vi "BuildArraySampleImages.vi"(11 "chaîne":string) -> (3 "3DArray":cluster{"Tableau":string[][]}[](array[cluster]))   [LabVIEW 2020]
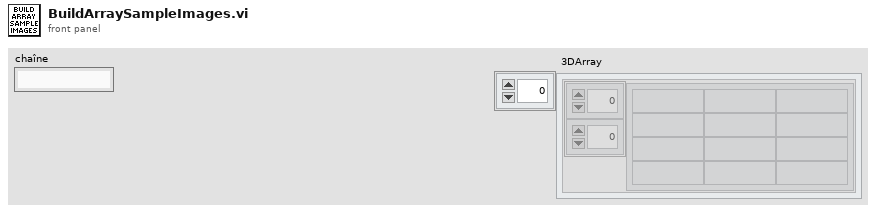
[diagram p1: front panel]
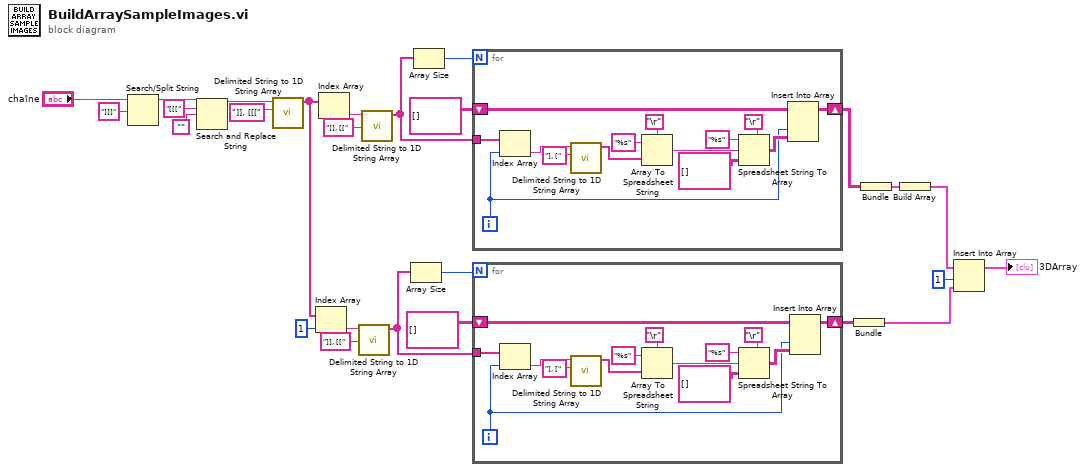
[diagram p0: block diagram]
diagram:
  n1 = Search/Split String(string="chaîne", search string/char (-)="]]]" ("chaîne/car. recherché (-)")) -> (substring before match=w25:string)  [unwired: 1 in, 2 out]
  n2 = Search and Replace String(input string=w25, search string="[[[" ("chaîne recherchée"), replace string="") -> (result string=w22:string)  [unwired: 5 in, 3 out]
  n3 = call <vilib>:"Delimited String to 1D String Array.vi"("delimiter"="]], [[[", "delimited string"=w22) -> ("string array"=w11:string[])  [unwired: 9 in]
  n4 = Index Array(array=w11, index=1 ("indice")) -> (element=w16:string)
  n5 = Index Array(array=w11) -> (element=w19:string)  [unwired: 1 in]
  n6 = call <vilib>:"Delimited String to 1D String Array.vi"("delimiter"="]], [[", "delimited string"=w16) -> ("string array"=w13:string[])  [unwired: 9 in]
  n7 = call <vilib>:"Delimited String to 1D String Array.vi"("delimiter"="]], [[", "delimited string"=w19) -> ("string array"=w18:string[])  [unwired: 9 in]
  n8 = Array Size(array=w13) -> (size(s)=w10:i32)
  n9 = Array Size(array=w18) -> (size(s)=w26:i32)
  n10 = for {
    N: w26 -> [_]
    tunnel: w18 -> [w40]
    shift-right: [w30] -> w9
    shift-left: string[][] [] -> [w31]
    i -> [w27]
    n11 = Index Array(array=w40, index=w27) -> (element=w35:string)
    n12 = call <vilib>:"Delimited String to 1D String Array.vi"("delimiter"="], [", "delimited string"=w35) -> ("string array"=w37:string[])  [unwired: 9 in]
    n13 = Array To Spreadsheet String(delimiter (Tab)="\r", array=w37, 3:"%s" ("chaîne de format")) -> (spreadsheet string=w32:string)
    n14 = Spreadsheet String To Array(delimiter (Tab)="\r", format string="%s" ("chaîne de format"), spreadsheet string=w32, array type (2D Dbl)=string[][] []) -> (array=w29:string[][])
    n15 = Insert Into Array(array=w31, index (col)=w27, new element=w29) -> (w30:string[][])  [unwired: 1 in]
  }
  n16 = for {
    N: w10 -> [_]
    tunnel: w13 -> [w54]
    shift-right: [w44] -> w8
    shift-left: string[][] [] -> [w45]
    i -> [w41]
    n17 = Index Array(array=w54, index=w41) -> (element=w49:string)
    n18 = call <vilib>:"Delimited String to 1D String Array.vi"("delimiter"="], [", "delimited string"=w49) -> ("string array"=w51:string[])  [unwired: 9 in]
    n19 = Array To Spreadsheet String(delimiter (Tab)="\r", array=w51, 3:"%s" ("chaîne de format")) -> (spreadsheet string=w46:string)
    n20 = Spreadsheet String To Array(delimiter (Tab)="\r", format string="%s" ("chaîne de format"), spreadsheet string=w46, array type (2D Dbl)=string[][] []) -> (array=w43:string[][])
    n21 = Insert Into Array(array=w45, index (col)=w41, new element=w43) -> (w44:string[][])  [unwired: 1 in]
  }
  n22 = Bundle(w8) -> (w5:cluster{string[][]})  [unwired: 1 in]
  n23 = Bundle(w9) -> (w7:cluster{string[][]})  [unwired: 1 in]
  n24 = Build Array(w7) -> (w6:cluster{string[][]}[])
  n25 = Insert Into Array(array=w6, index=1 ("indice"), new element=w5) -> (→"3DArray":cluster{string[][]}[])
